vi "Lockin.Engine.vi"(8 "error in (no error)":errorcluster, 11 "Instrument.DAQ":refnum<class "Instrument.DAQ.lvclass">) -> (0 "error out":errorcluster, 1 "SweepResults":T1, 2 "<Results> (X,Y,R,Theta,Mean)":T2 {"Results (Dictionary)"."value" format="%#_6p"}, 3 "Instrument.DAQ out":refnum<class "Instrument.DAQ.lvclass">)   [LabVIEW 2019, in "Instrument.DAQ.lvclass"]
uses:
  Instrument.DAQ.lvclass
  Typedefs/Results--Cluster.ctl
  Instrument.DAQ.lvclass/Instrument.DAQ.ctl
  <vilib>/Analysis/baseanly.llb/Mean (DBL).vi
  <vilib>/Analysis/NI_AALBase.lvlib
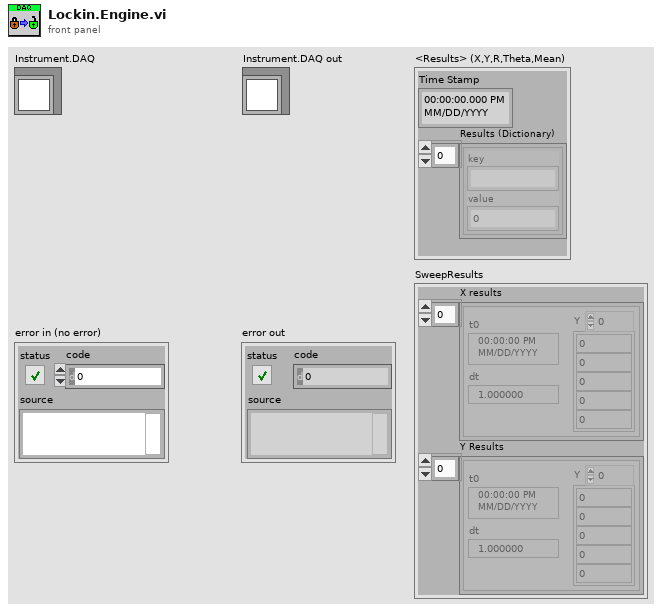
[diagram p1: front panel]
types:
  T1 = cluster{"X results":waveform(dbl)[], "Y Results":waveform(dbl)[]}
  T2 = typedef "Instrument.DAQ.lvclass/Results--Cluster.ctl" = cluster{"Time Stamp":timestamp, "Results (Dictionary)":cluster{"key":string, "value":dbl}[]}
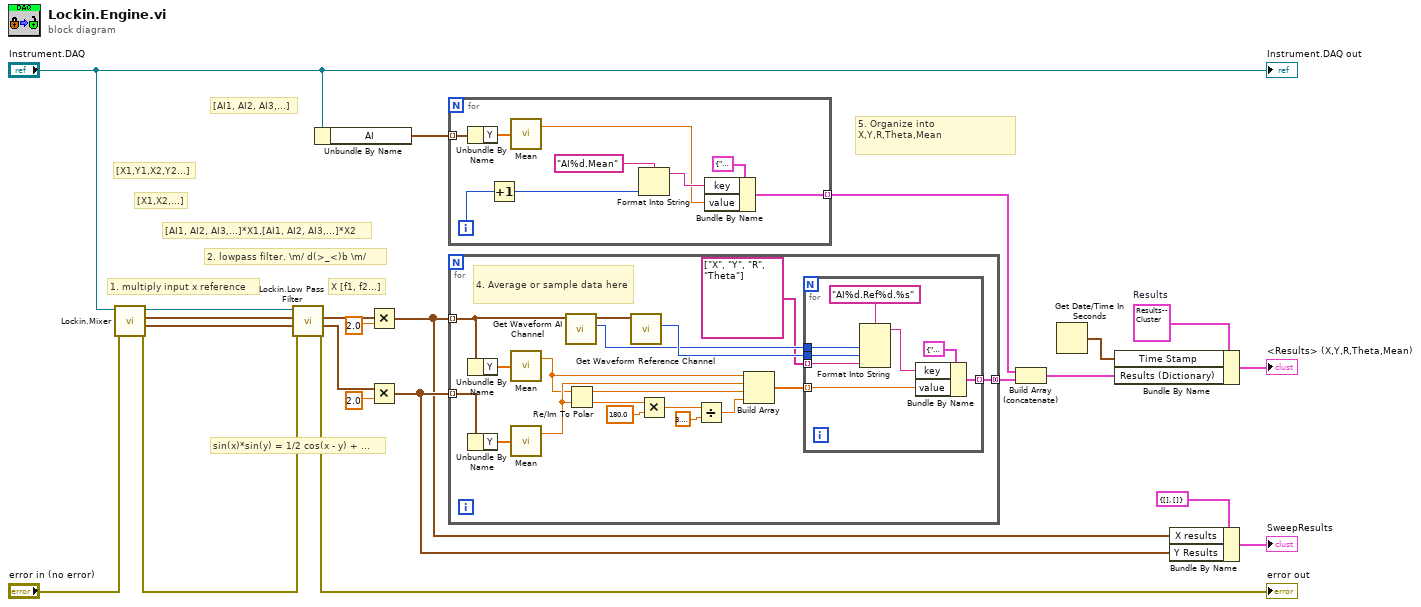
[diagram p0: block diagram]
diagram:
  w22 = T2 {"Time Stamp"=timestamp(0 s since 1904-01-01), "Results (Dictionary)"=[]}  # Results
  # "sin(x)*sin(y) = 1/2 cos(x - y) + ..."
  # "[X1,X2,...]"
  # "1. multiply input x reference"
  # "X [f1, f2...]"
  # "2. lowpass filter. \\m/ d(>_<)b \\m/"
  # "[AI1, AI2, AI3,...]*X1,[AI1, AI2, AI3,...]*X2"
  # "[AI1, AI2, AI3,...]"
  # "[X1,Y1,X2,Y2...]"
  # "5. Organize into X,Y,R,Theta,Mean"
  n1 = call "Lockin.Mixer.vi"("error in (no error)"="error in (no error)", "Instrument.DAQ"="Instrument.DAQ") -> ("error out"=w1:errorcluster, "Y out"=w5:waveform(dbl)[], "X out"=w16:waveform(dbl)[], "Instrument.DAQ"=w20:refnum<class "Instrument.DAQ.lvclass">)  [unwired: 6 in]
  n2 = call "Lockin.Low Pass Filter.vi"("error in (no error)"=w1, "Y"=w5, "X"=w16, "Lockin.DAQ"=w20) -> ("error out"=→"error out":errorcluster, "Y out"=w3:waveform(dbl)[], "X out"=w4:waveform(dbl)[])  [unwired: 4 in, 1 out]
  n3 = Unbundle By Name("Instrument.DAQ") -> ("AI"=w6:waveform(dbl)[])
  n4 = Multiply(x=w4, y=2.0) -> (x*y=w12:waveform(dbl)[])
  n5 = Multiply(x=w3, y=2.0) -> (x*y=w13:waveform(dbl)[])
  n6 = for {
    tunnel: w6 -> [w31] mode=indexing
    tunnel: [w25] -> w9 mode=indexing
    i -> [w24]
    n7 = Unbundle By Name(w31) -> ("Y"=w30:dbl[])
    n8 = Increment(x=w24) -> (x+1=w23:i32)
    n9 = call-poly <vilib>:"Mean.vi"("X"=w30) -> ("mean"=w26:dbl)  [unwired: 1 out]
    n10 = Format Into String(format string="AI%d.Mean", w23) -> (resulting string=w28:string)  [unwired: 2 in, 1 out]
    n11 = Bundle By Name(cluster=cluster{"key":string, "value":dbl} {"key"="", "value"=0.0} ("key-value"), "key"=w28, "value"=w26) -> (w25:cluster{"key":string, "value":dbl})
  }
  n12 = for {
    tunnel: w12 -> [w34] mode=indexing
    tunnel: w13 -> [w33] mode=indexing
    tunnel: [w38] -> w10 mode=concatenating
    # "4. Average or sample data here"
    n13 = Unbundle By Name(w34) -> ("Y"=w43:dbl[])
    n14 = Unbundle By Name(w33) -> ("Y"=w42:dbl[])
    n15 = call-poly <vilib>:"Mean.vi"("X"=w43) -> ("mean"=w40:dbl)  [unwired: 1 out]
    n16 = call-poly <vilib>:"Mean.vi"("X"=w42) -> ("mean"=w41:dbl)  [unwired: 1 out]
    n17 = call "Get Waveform AI Channel.vi"("Reference in"=w34) -> ("AI Channel"=w35:i32, "Reference out"=w39:waveform(dbl))  [unwired: 8 in, 1 out]
    n18 = Re/Im To Polar(2:w41, 3:w40) -> (0:w46:dbl, 1:w44:dbl)
    n19 = call "Get Waveform Reference Channel.vi"("Reference in"=w39) -> ("Reference Channel"=w36:i32)  [unwired: 8 in, 2 out]
    n20 = Multiply(x=w46, y=180.0) -> (x*y=w45:dbl)
    n21 = Divide(x=w45, y=3.141592653589793) -> (x/y=w49:dbl)
    n22 = Build Array(w40, w41, w44, w49) -> (w37:dbl[])
    n23 = for {
      tunnel: w37 -> [w57] mode=indexing
      tunnel: string[] ["X", "Y", "R", "Theta"] -> [w51] mode=indexing
      tunnel: [w55] -> w38 mode=indexing
      tunnel: w36 -> [w52]
      tunnel: w35 -> [w54]
      n24 = Format Into String(format string="AI%d.Ref%d.%s", w54, w52, w51) -> (resulting string=w50:string)  [unwired: 2 in, 1 out]
      n25 = Bundle By Name(cluster=cluster{"key":string, "value":dbl} {"key"="", "value"=0.0} ("key-value"), "key"=w50, "value"=w57) -> (w55:cluster{"key":string, "value":dbl})
    }
  }
  n26 = Build Array (concatenate)(w9, w10) -> (w8:cluster{"key":string, "value":dbl}[])
  n27 = Get Date/Time In Seconds() -> (seconds since 1Jan1904=w2:timestamp)
  n28 = Bundle By Name(cluster=w22, "Time Stamp"=w2, "Results (Dictionary)"=w8) -> (→"<Results> (X,Y,R,Theta,Mean)":T2)
  n29 = Bundle By Name(cluster=T1 {"X results"=[], "Y Results"=[]} ("SweepResults"), "X results"=w12, "Y Results"=w13) -> (→"SweepResults":T1)
  "Instrument.DAQ out" <- "Instrument.DAQ"
